vi "SCISCAN Image display TO Enum .vi"(7 "SCISCAN Image display_to_Enum_Commands":T2, 8 "Error In":errorcluster, 11 "UI control refnums":T1) -> (0 "Error Out":errorcluster)   [LabVIEW 2012]
doc: "SciScan 1.2 160622"
uses:
  SCISCAN Image display to Enum_Commands.ctl
  Custom Controls and Typedefs/Macro_MD_UI Control Refnums.ctl
  Custom Controls and Typedefs/Delete Button.ctl
  Custom Controls and Typedefs/Edit Button.ctl
  Custom Controls and Typedefs/Timing Estimate Cluster.ctl
  CommonResource VIs/Timing/Timing Indicator.ctl
  Custom Controls and Typedefs/Load from PSM Button.ctl
  Custom Controls/MAIN Image panel reso tab Control type def.ctl
  Custom Controls/MAIN Image panel tab Control type def.ctl
  GFG/GFGfpRefGet.vi
  GFG/GFG library.lvlib
panel:
  # "(hh:mm:ss)"
  # "(hh:mm:ss)"
  # "(hh:mm:ss)"
  # "(hh:mm:ss)"
  # "(hh:mm:ss)"
  # "(hh:mm:ss)"
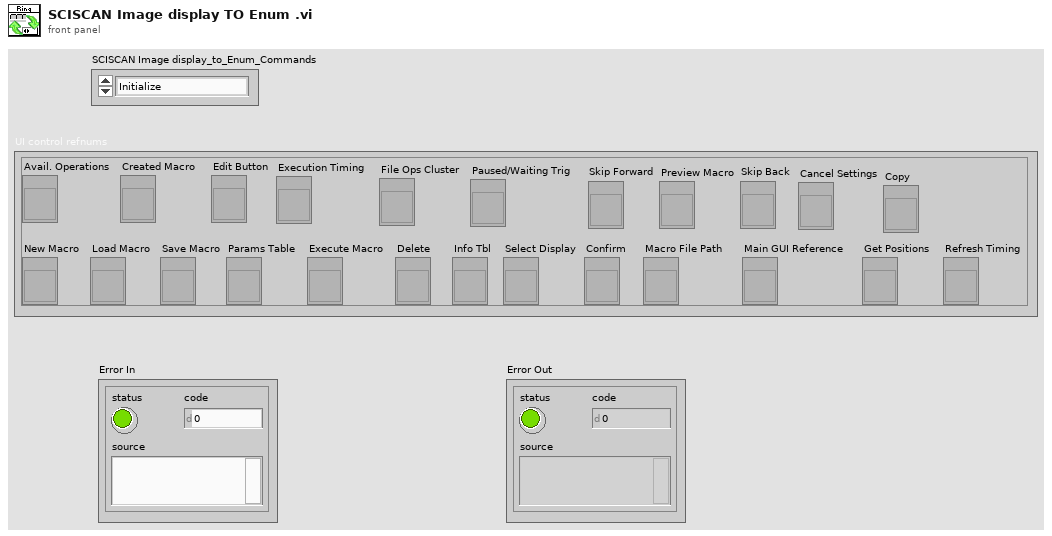
[diagram p1: front panel]
types:
  T1 = typedef "Macro_MD_UI Control Refnums.ctl" = cluster{"Avail. Operations":refnum<vi>, "Created Macro":refnum<vi>, "Load Macro":refnum<vi>, "Save Macro":refnum<vi>, "Params Table":refnum<vi>, "Delete":refnum<vi>, "Edit Button":refnum<vi>, "Execute Macro":refnum<vi>, "Info Tbl":refnum<vi>, "Execution Timing":refnum<vi>, "Select Display":refnum<vi>, "File Ops Cluster":refnum<vi>, "Paused/Waiting Trig":refnum<vi>, "Confirm":refnum<vi>, "New Macro":refnum<vi>, "Preview Macro":refnum<vi>, "Skip Forward":refnum<vi>, "Skip Back":refnum<vi>, "Macro File Path":refnum<vi>, "Main GUI Reference":refnum<vi>, "Cancel Settings":refnum<vi>, "Get Positions":refnum<vi>, "Copy":refnum<vi>, "Refresh Timing":refnum<vi>}
  T2 = typedef "SCISCAN Image display to Enum_Commands.ctl" = enum16{"Initialize", "SCISCAN disp to Enum", "Enum to SCISCAN disp"}
  T3 = typedef "MAIN Image panel tab Control type def.ctl" = enum32{"Channel 1", "Channel 2", "Channel 3", "Channel 4", "all channels", "RGB overlay", "ROI", "arbitrary line scan"}
  T4 = typedef "MAIN Image panel reso tab Control type def.ctl" = enum32{"Channel 1", "Channel 2", "Channel 3", "Channel 4", "Channel 5", "all channels", "RGB overlay", "ROI", "arbitrary line scan"}
  T5 = cluster{"WaveformChartRef":refnum<vi>, "DigitalRef":refnum<vi>, "ArrayRef":refnum<vi>, "TabControlRef":refnum<vi>, "EnumRef":refnum<vi>, "RingRef":refnum<vi>, "BooleanRef":refnum<vi>, "KnobRef":refnum<vi>, "SlideRef":refnum<vi>, "PathRef":refnum<vi>, "StringRef":refnum<vi>, "ComboBox":refnum<vi>, "WaveformGraphRef":refnum<vi>}
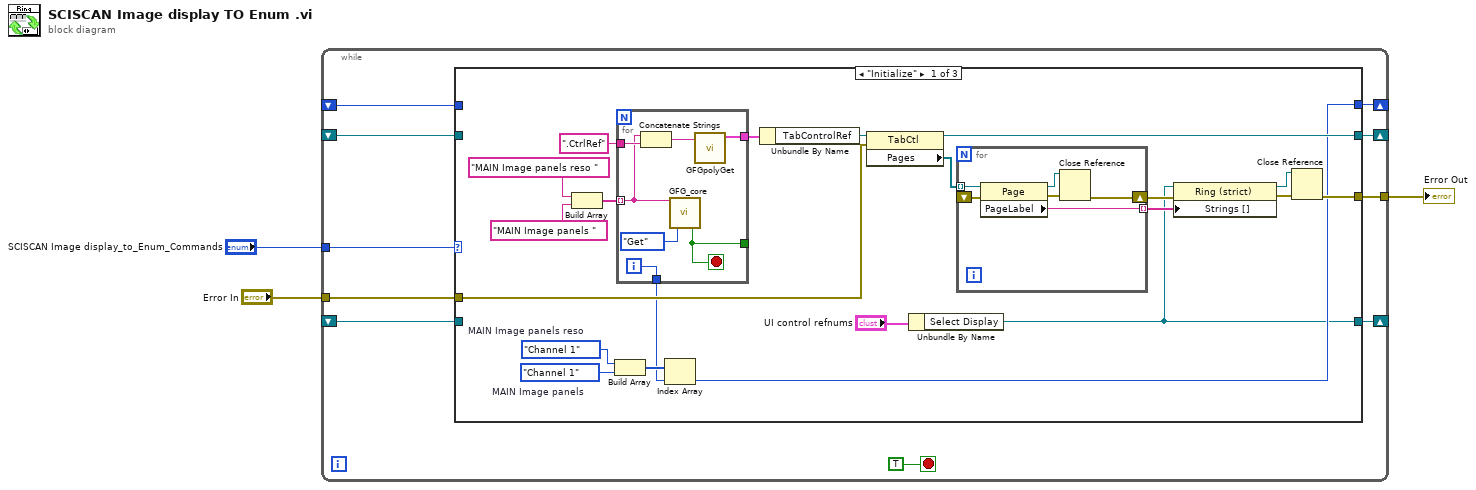
[diagram p0: block diagram]
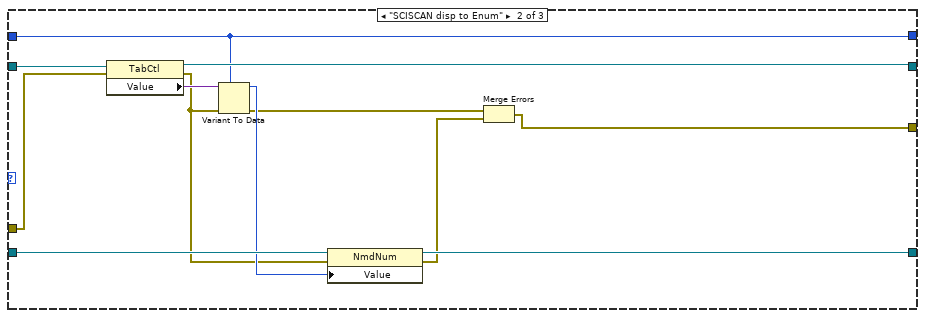
[diagram p2: hidden frame]
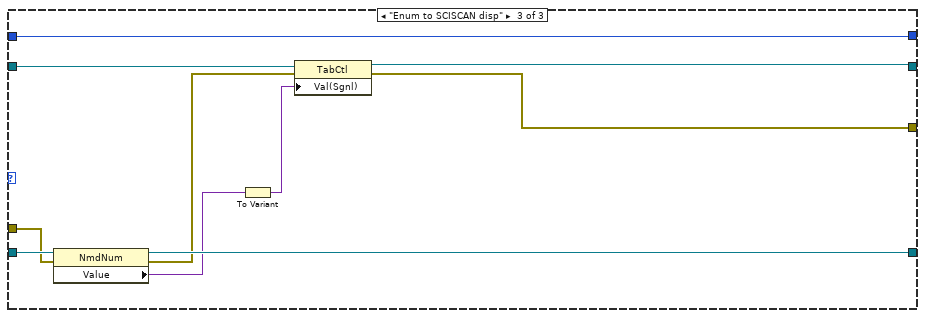
[diagram p3: hidden frame]
diagram:
  n1 = while {
    tunnel: "SCISCAN Image display_to_Enum_Commands" -> [w13]
    shift-right: [w11] -> _
    shift-left: _ -> [w10]
    shift-right: [w8] -> _
    shift-left: _ -> [w9]
    tunnel: [w7] -> w2
    tunnel: "Error In" -> [w6]
    shift-right: [w5] -> _
    shift-left: _ -> [w4]
    stop <- TRUE stop-if-true
    n2 = case shown="\"Initialize\"" w13 {
      tunnel: [w28 w51 w66] -> w11
      tunnel: w10 -> [_ w58 w69]
      tunnel: w9 -> [_ w57 w68]
      tunnel: [w14 w54 w67] -> w8
      tunnel: [w21 w48 w60] -> w7
      tunnel: w6 -> [w20 w56 w62]
      tunnel: [w15 w50 w65] -> w5
      tunnel: w4 -> [_ w50 w65]
      frame "Initialize" {
        w18 = MAIN_Image_panel_tab_Control_type_def."Channel 1"  # MAIN Image panels
        w19 = MAIN_Image_panel_reso_tab_Control_type_def."Channel 1"  # MAIN Image panels reso
        n3 = Build Array("MAIN Image panels reso " ("Tip Strip"), "MAIN Image panels " ("Tip Strip")) -> (w32:string[])
        n4 = Build Array(w19, w18) -> (w17:u32[])
        n5 = for {
          tunnel: w32 -> [w44] mode=indexing
          tunnel: [w46] -> _
          tunnel: ".CtrlRef" ("Tip Strip") -> [w45]
          tunnel: [w42] -> w30
          tunnel: [w41] -> w16
          i -> [w41]
          stop <- w46 stop-if-true
          n6 = Concatenate Strings(w44, w45) -> (w43:string)
          n7 = call "GFG_core.vi"("Variable Name in"=w44, "Action"=enum16{"Init", "Set", "Get", "Clear"}."Get") -> ("Found/Replaced"=w46:bool)  [unwired: 11 in, 6 out]
          n8 = call-poly "GFGpolyGet.vi"("Variable Name in"=w43) -> ("output cluster"=w42:T5)  [unwired: 9 in, 1 out]
        }
        n9 = Index Array(array=w17, index=w16) -> (element=w15:u32)
        n10 = Unbundle By Name(w30) -> ("TabControlRef"=w29:refnum<vi>)
        n11 = property class="TabCtl"(reference=w29, error in=w20) -> (reference out=w28:refnum<vi>, "Pages"=w27:refnum<vi>[])  [unwired: 1 out]
        n12 = Unbundle By Name("UI control refnums") -> ("Select Display"=w14:refnum<vi>)
        n13 = for {
          tunnel: w27 -> [w40] mode=indexing
          shift-right: [w37] -> w24
          shift-left: _ -> [w36]
          tunnel: [w35] -> w25 mode=indexing
          n14 = property class="Page"(reference=w40, error in=w36) -> (reference out=w38:refnum<vi>, error out=w39:errorcluster, "PageLabel"=w35:string)
          n15 = Close Reference(reference=w38, error in (no error)=w39) -> (error out=w37:errorcluster)
        }
        n16 = property class="Ring (strict)"(reference=w14, error in=w24, "Strings []"=w25) -> (reference out=w22:refnum<vi>, error out=w23:errorcluster)
        n17 = Close Reference(reference=w22, error in (no error)=w23) -> (error out=w21:errorcluster)
      }
      frame "SCISCAN disp to Enum" {
        n18 = property class="TabCtl"(reference=w58, error in=w56) -> (reference out=w51:refnum<vi>, error out=w53:errorcluster, "Value"=w59:variant)
        n19 = Variant To Data(error in=w53, type=w50, Variant=w59) -> (data=w55:u32, error out=w52:errorcluster)
        n20 = property class="NmdNum"(reference=w57, error in=w53, "Value"=w55) -> (reference out=w54:refnum<vi>, error out=w49:errorcluster)
        n21 = Merge Errors(w52, w49) -> (w48:errorcluster)
      }
      frame "Enum to SCISCAN disp" {
        n22 = property class="NmdNum"(reference=w68, error in=w62) -> (reference out=w67:refnum<vi>, error out=w61:errorcluster, "Value"=w64:variant)
        n23 = To Variant(anything=w64) -> (Variant=w63:variant)
        n24 = property class="TabCtl"(reference=w69, error in=w61, "Val(Sgnl)"=w63) -> (reference out=w66:refnum<vi>, error out=w60:errorcluster)
      }
    }
  }
  "Error Out" <- w2
